vi "RP100IDnQuery.vi"(2 "error in (no error)":errorcluster, 3 "VISA resource name":refnum<visa-resource-name>) -> (0 "error out":errorcluster, 1 "VISA resource name out":refnum<visa-resource-name>)   [LabVIEW 2020]
uses:
  <vilib>/regexp/Match Regular Expression.xnode
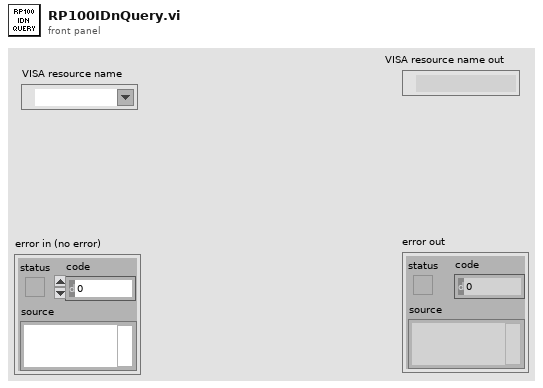
[diagram p1: front panel]
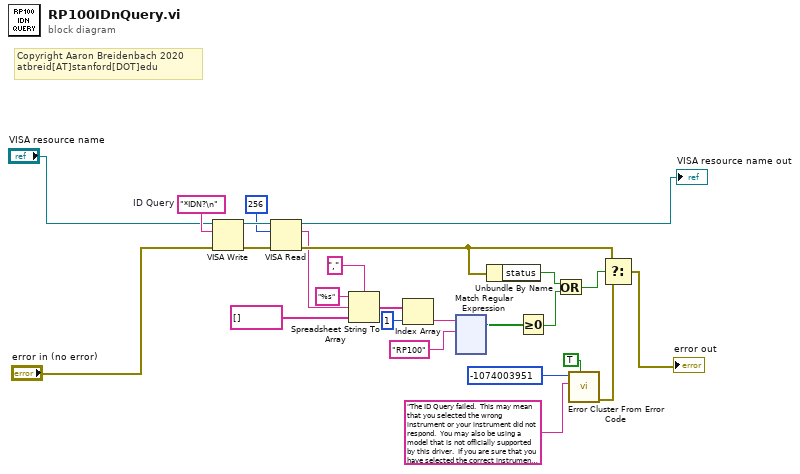
[diagram p0: block diagram]
diagram:
  w22 = "*IDN?\n"  # ID Query
  # "Copyright Aaron Breidenbach 2020\natbreid[AT]stanford[DOT]edu"
  n1 = VISA Write(VISA resource name="VISA resource name", write buffer=w22, error in (no error)="error in (no error)") -> (VISA resource name out=w25:refnum<visa-resource-name>, error out=w24:errorcluster)  [unwired: 1 out]
  n2 = VISA Read(VISA resource name=w25, byte count=u32 256, error in (no error)=w24) -> (VISA resource name out=→"VISA resource name out":refnum<visa-resource-name>, read buffer=w13:string, error out=w17:errorcluster)  [unwired: 1 out]
  n3 = Spreadsheet String To Array(delimiter (Tab)=",", format string="%s", spreadsheet string=w13, array type (2D Dbl)=string[] []) -> (array=w11:string[])
  n4 = Index Array(array=w11, index=1) -> (element=w7:string)
  n5 = xnode "Match Regular Expression"("input string"=w7, "regular expression"="RP100") -> ("offset past match"=w5:i32)  [unwired: 4 in, 4 out]
  n6 = Unbundle By Name(w17) -> ("status"=w16:bool)
  n7 = Greater Or Equal To 0?(x=w5) -> (x >= 0?=w6:bool)
  n8 = Or(x=w16, y=w6) -> (x .or. y?=w15:bool)
  n9 = call <vilib>:"Error Cluster From Error Code.vi"("show call chain? (False)"=TRUE, "error message (\"\")"="The ID Query failed.  This may mean that you selected the wrong instrument or your instrument did not respond.  You may also be using a model that is not officially supported by this driver.  If you are sure that you have selected the correct instrument and it is responding, try disabling the ID Query." ("Source (VI Name)"), "error code (0)"=-1074003951 ("Code")) -> ("error out"=w21:errorcluster)  [unwired: 6 in]
  n10 = Select(t=w17, s=w15, f=w21) -> (s? t:f=→"error out":errorcluster)
